vi "get Current Path.vi"(11 "Log in":refnum<class "Log.lvclass">) -> (3 "Current Path":path)   [LabVIEW 2020, in "Log.lvclass"]
uses:
  Log.lvclass
  Log.lvclass/Log.ctl
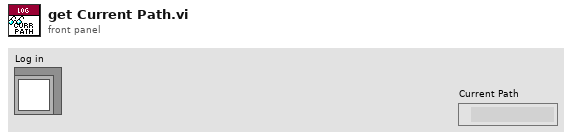
[diagram p1: front panel]
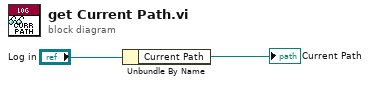
[diagram p0: block diagram]
diagram:
  n1 = Unbundle By Name("Log in") -> ("Current Path"=→"Current Path":path)
